vi "Test-DeviceInit.vi"(4 "ConfigData":string, 5 "DeviceName":string) -> (0 "InitOK?":bool, 1 "DeviceData":T1, 2 "VI Refnum":refnum<vi>)   [LabVIEW 2019]
uses:
  <vilib>/Utility/error.llb/DialogType.ctl
panel:
  out "KeyFind?":bool[](array[boolean])
  out "KeyValues":string[](array[string])
  out "DeviceID":string
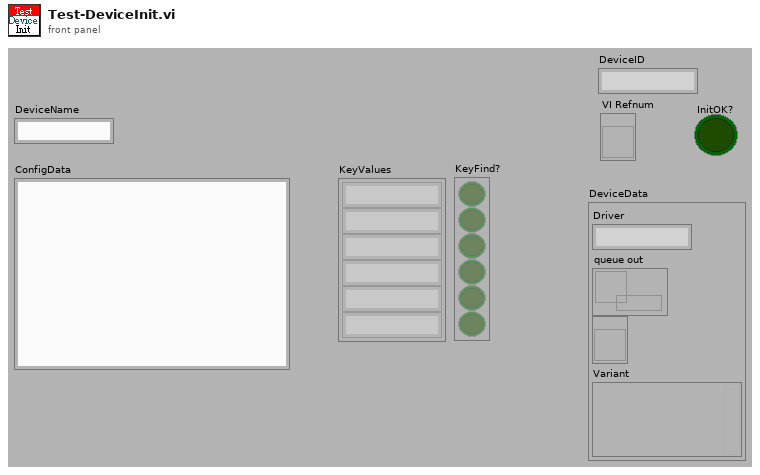
[diagram p1: front panel]
types:
  T1 = cluster{"Driver":string, "queue out":refnum<queue>, refnum<vi>, "Variant":variant}
  T2 = cluster{"Command":string, "Parameter":string, "queue out":refnum<queue>}
  T3 = typedef "DialogType.ctl" = u16
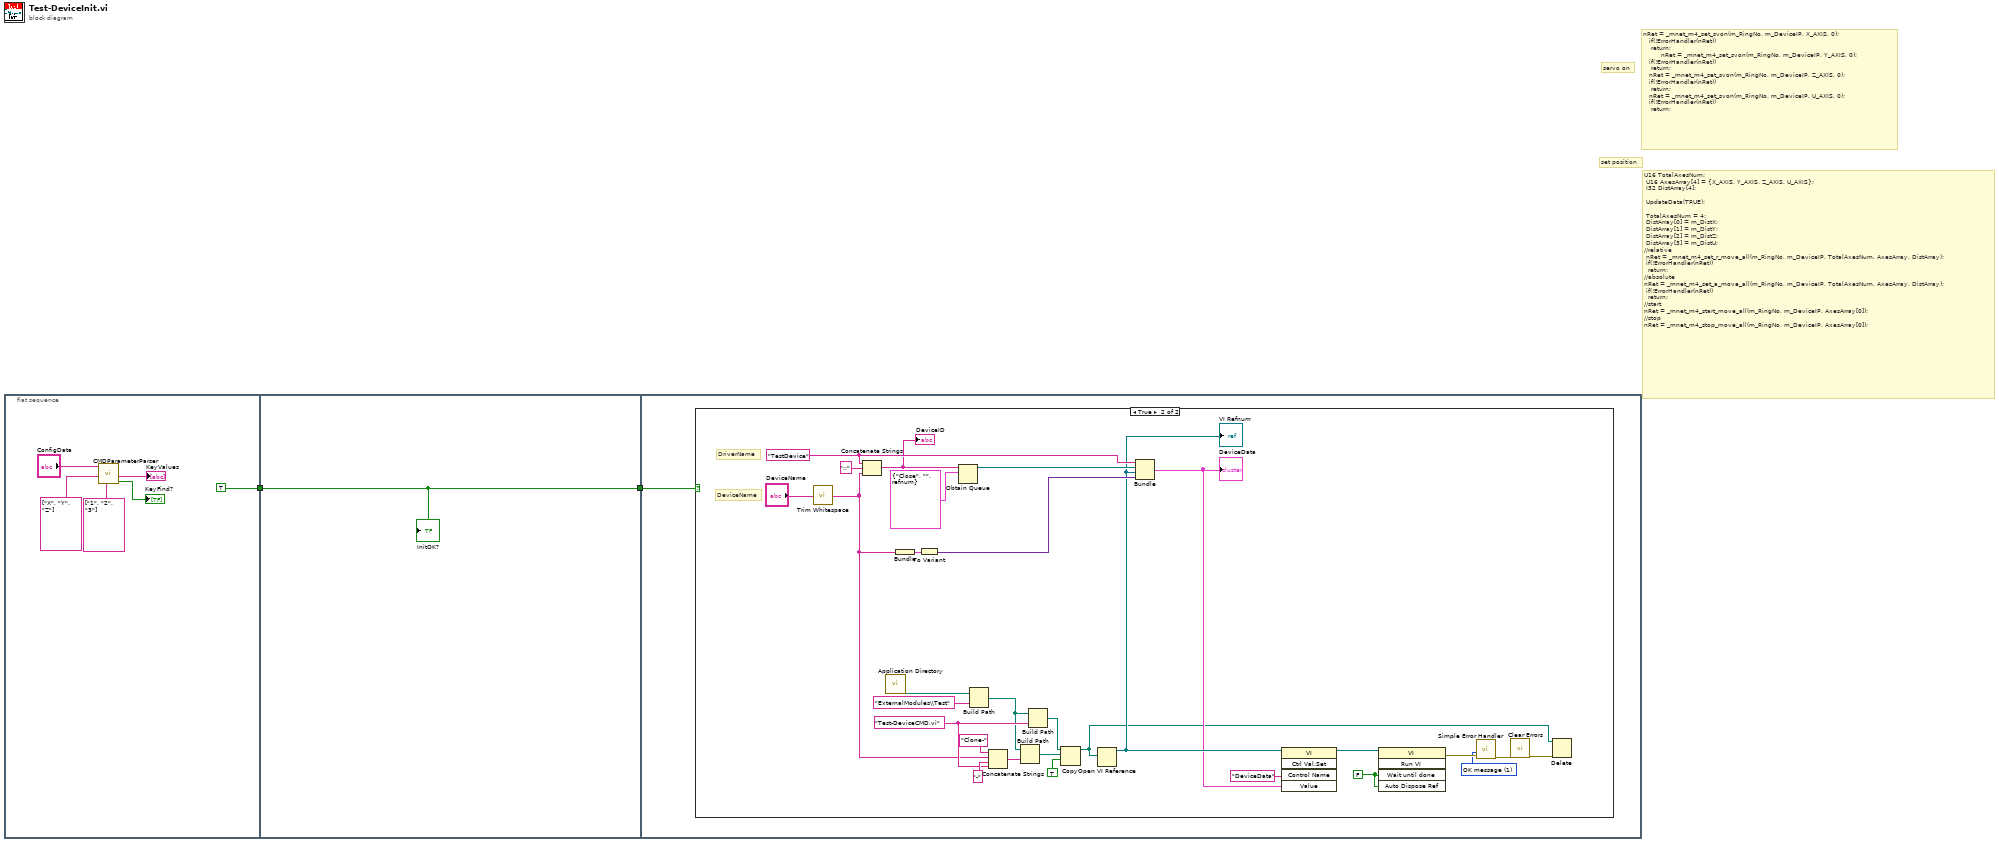
[diagram p0: block diagram]
diagram:
  # "set position"
  # "U16 TotalAxesNum;\n\tU16 AxesArray[4] = {X_AXIS, Y_AXIS, Z_AXIS, U_AXIS};\n\tI32 DistArray[4];\n\n\tUpdateData(TRUE);\n\n\tTotalAxesNum = 4;\n\tDistArray[0] = m_DistX;\n\tDistArray[1] = m_DistY;\n\tDistArray[2] = m_DistZ;\n\tDistArray[3] = m_DistU;\n//relative\n\tnRet = _mnet_m4_set_r_move_all(m_RingNo, m_DeviceIP, TotalAxesNum, AxesArray, DistArray);\n\tif(!ErrorHandler(nRet))\n\t\treturn;\n//absolute\nnRet = _mnet_m4_set_a_move_all(m_RingNo, m_DeviceIP, TotalAxesNum, AxesArray, DistArray);\n\tif(!ErrorHandler(nRet))\n\t\treturn;\n//start\nnRet = _mnet_m4_start_move_all(m_RingNo, m_DeviceIP, AxesArray[0]);\n//stop\nnRet = _mnet_m4_stop_move_all(m_RingNo, m_DeviceIP, AxesArray[0]);"
  # "servo on"
  # "nRet = _mnet_m4_set_svon(m_RingNo, m_DeviceIP, X_AXIS, 0);\n\t\t if(!ErrorHandler(nRet))\n\t\t\t return;\n         nRet = _mnet_m4_set_svon(m_RingNo, m_DeviceIP, Y_AXIS, 0);\n\t\t if(!ErrorHandler(nRet))\n\t\t\t return;\n\t\t nRet = _mnet_m4_set_svon(m_RingNo, m_DeviceIP, Z_AXIS, 0);\n\t\t if(!ErrorHandler(nRet))\n\t\t\t return;\n\t\t nRet = _mnet_m4_set_svon(m_RingNo, m_DeviceIP, U_AXIS, 0);\n\t\t if(!ErrorHandler(nRet))\n\t\t\t return;"
  n1 = flat-sequence {
    tunnel: [TRUE] -> w1
    tunnel: [w9] -> w2
    tunnel: w1 -> [w9]
    tunnel: w2 -> [w10]
    frame #0 {
      n2 = call "CMDParameterParser.vi"("DeafultValues"=string[] ["1", "2", "3"] ("ParameterKey"), "RequiredKeys"=string[] ["X", "Y", "Z"] ("ParameterKey"), "CMDParameter"="ConfigData") -> ("KeyFind?"=→"KeyFind?":bool[], "KeyValues"=→"KeyValues":string[])  [unwired: 6 in, 1 out]
    }
    frame #1 {
      "InitOK?" <- w9
    }
    frame #2 {
      n3 = case shown="True" w10 {
        frame False {
        }
        frame True {
          w14 = T3 1 items=["no dialog", "OK message", "continue or stop message", "OK message + warnings", "continue/stop + warnings"] ("type of dialog (OK msg:1)")
          w29 = FALSE ("Wait Until Done")
          w33 = "Test-DeviceCMD.vi" ("name or relative path")
          w23 = "TestDevice" ("Driver")
          # "DeviceName"
          # "DriverName"
          n4 = call <vilib>:"Trim Whitespace.vi"("string"="DeviceName") -> ("trimmed string"=w17:string)  [unwired: 1 in]
          n5 = Concatenate Strings(w23, "::" ("string"), w17) -> (w21:string)
          "DeviceID" <- w21
          n6 = call <vilib>:"Application Directory.vi"() -> ("Application Directory"=w25:path)
          n7 = Bundle("trimmed string"=w17) -> (w39:cluster{"trimmed string":string})  [unwired: 1 in]
          n8 = To Variant(anything=w39) -> (Variant=w26:variant)
          n9 = Obtain Queue(name (unnamed)=w21, element data type=T2 {"Command"="Close", "Parameter"="", "queue out"=refnum} ("Motor Module CMD")) -> (queue out=w30:refnum<queue>)  [unwired: 3 in, 2 out]
          n10 = Build Path(base path=w25, name or relative path="ExternalModules\\Test") -> (appended path=w16:path)
          n11 = Concatenate Strings("Clone-" ("string"), w17, "-" ("string"), w33) -> (w37:string)
          n12 = Build Path(base path=w16, name or relative path=w37) -> (appended path=w35:path)
          n13 = Build Path(base path=w16, name or relative path=w33) -> (appended path=w32:path)
          n14 = Copy(9:TRUE ("overwrite (F)"), 10:w35, 11:w32) -> (3:w11:path)  [unwired: 2 in, 2 out]
          n15 = Open VI Reference(vi path=w11) -> (vi reference=w19:refnum<vi>)  [unwired: 5 in, 1 out]
          "VI Refnum" <- w19
          n16 = Bundle("Driver"=w23, "queue out"=w30, w19, "Variant"=w26) -> (w18:T1)  [unwired: 1 in]
          "DeviceData" <- w18
          n17 = invoke class="VI" method="Ctrl Val.Set"(reference=w19, "Control Name"="DeviceData", "Value"=w18) -> (reference out=w20:refnum<vi>)  [unwired: 2 in, 4 out]
          n18 = invoke class="VI" method="Run VI"(reference=w20, "Wait until done"=w29, "Auto Dispose Ref"=w29) -> (error out=w15:errorcluster)  [unwired: 2 in, 4 out]
          n19 = call <vilib>:"Simple Error Handler.vi"("type of dialog (OK msg:1)"=w14, "error in (no error)"=w15) -> ("error out"=w13:errorcluster)  [unwired: 3 in, 4 out]
          n20 = call <vilib>:"Clear Errors.vi"("error in (no error)"=w13) -> ("error out"=w12:errorcluster)  [unwired: 5 in, 1 out]
          n21 = Delete(path (use dialog)=w11, error in=w12) -> ()  [unwired: 3 in, 3 out]
        }
      }
    }
  }
